vi "host.vi"() -> ()   [LabVIEW 2020]
uses:
  <vilib>/FPGAPlugInAG/cRIO-9035/niLvFpga_Open_cRIO-9035.vi
  <vilib>/rvi/interface/common/dynamic/niFpgaDynamicAddResources.vi
  <vilib>/Utility/error.llb/Error Cluster From Error Code.vi
  <vilib>/rvi/errors/niLvFpgaAdjustHostInterfaceError.vi
  <vilib>/FPGAPlugInAG/Dynamic/niLvFpga_Run_Dynamic.vi
  <vilib>/FPGAPlugInAG/Dynamic/niLvFpga_Close_Dynamic.vi
  <vilib>/rvi/interface/nirviOpenFPGA/nirviOpenFPGA.xnode
  FPGA Bitfiles/v1.2_FPGATarget_target_ruB+bBOu3LI.lvbitx
  target.vi
  <vilib>/rvi/interface/nirviMethod/nirviMethod.xnode
  <vilib>/rvi/interface/nirviReadWriteControl/nirviReadWriteControl.xnode
  <vilib>/rvi/interface/nirviCloseFPGA/nirviCloseFPGA.xnode
  <vilib>/rvi/errors/niLvFpgaMergeErrorWithErrorCode.vi
  <vilib>/FPGAPlugInAG/Dynamic/niLvFpga_WriteFifo_Dynamic.vi
  <vilib>/FPGAPlugInAG/Dynamic/niLvFpga_ReadFifo_Dynamic.vi
  NiFpgaLv.dll
  <vilib>/rvi/interface/Simulation/niFpgaSimulationCallBeginRW.vi
panel:
  out "transposed array":fxp<+/-,32,16>[][](array[numeric])
  out "output array":fxp<+/-,32,16>[][](array[numeric])
  out "n out":i32
  out "m out":i32
  out "sum of error":dbl
  out "B - FPGA code":sgl[][](array[numeric])
  out "A":sgl[][](array[numeric])
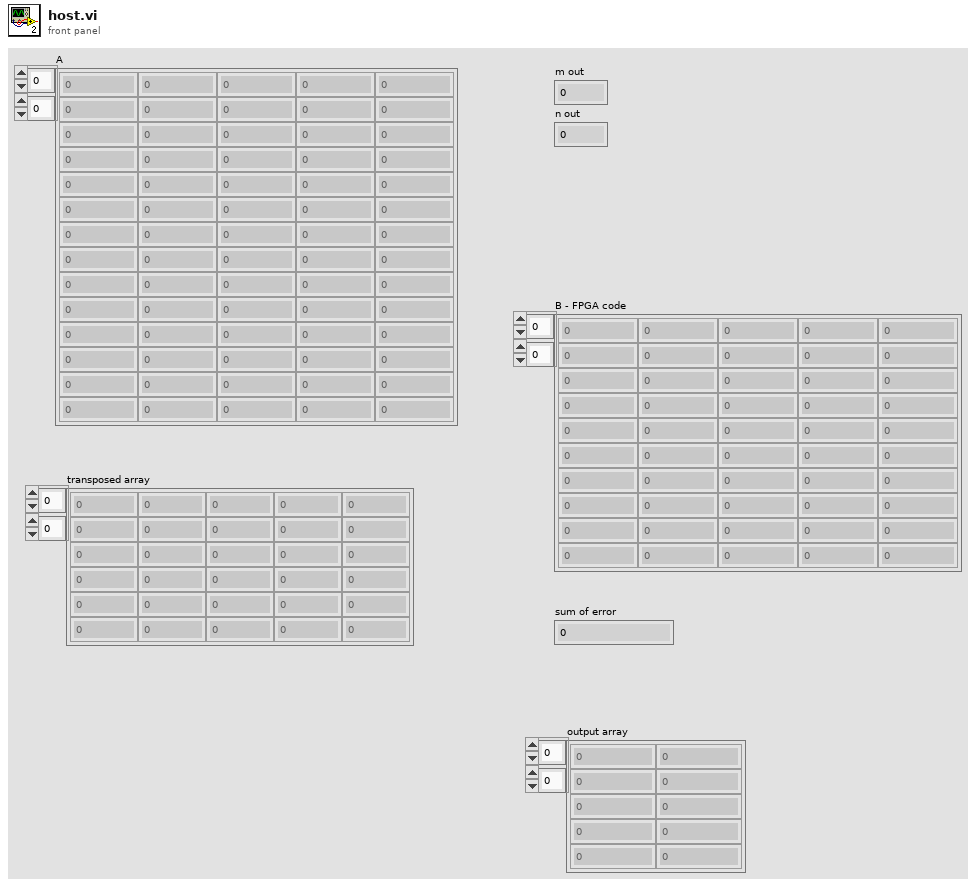
[diagram p1: front panel]
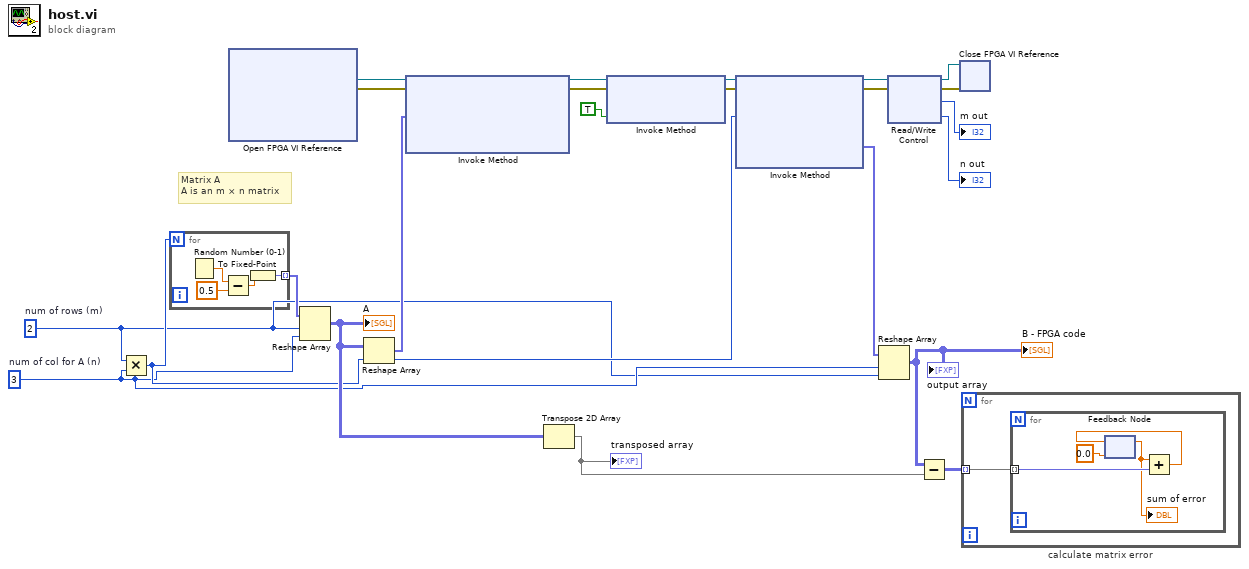
[diagram p0: block diagram]
diagram:
  w8 = 3  # num of col for A (n)
  w7 = 2  # num of rows (m)
  # "Matrix A\nA is an m × n matrix"
  n1 = Multiply(x=w7, y=w8) -> (x*y=w12:i32)
  n2 = for {
    N: w12 -> [_]
    tunnel: [w25] -> w18 mode=indexing
    n3 = Random Number (0-1)() -> (number: 0 to 1=w27:dbl)
    n4 = Subtract(x=w27, y=sgl 0.5) -> (x-y=w24:sgl)
    n5 = To Fixed-Point(number=w24) -> (fixed-point=w25:fxp<+/-,32,16>)  [unwired: 1 in]
  }
  n6 = xnode "Open FPGA VI Reference"() -> ("FPGA VI Reference Out"=w22:refnum<k20>, "error out"=w21:errorcluster)  [unwired: 2 in]
  n7 = Reshape Array(w18, w7, w8) -> (w14:fxp<+/-,32,16>[][])
  "A" <- w14
  n8 = Reshape Array(w14, w12) -> (w17:fxp<+/-,32,16>[])
  n9 = xnode "Invoke Method"("FPGA VI Reference In"=w22, "error in"=w21, "Data"=w17) -> ("FPGA VI Reference Out"=w11:refnum<k20>, "error out"=w10:errorcluster)  [unwired: 1 in, 1 out]
  n10 = Transpose 2D Array(2D array=w14) -> (transposed array=w13:fxp<+/-,32,16>[][])
  "transposed array" <- w13
  n11 = xnode "Invoke Method"("FPGA VI Reference In"=w11, "error in"=w10, "Wait Until Done (F)"=TRUE) -> ("FPGA VI Reference Out"=w20:refnum<k20>, "error out"=w19:errorcluster)
  n12 = xnode "Invoke Method"("FPGA VI Reference In"=w20, "error in"=w19, "Number of Elements"=w12) -> ("FPGA VI Reference Out"=w6:refnum<k20>, "error out"=w2:errorcluster, "Data"=w15:fxp<+/-,32,16>[])  [unwired: 1 in, 1 out]
  n13 = Reshape Array(w15, w8, w7) -> (w9:fxp<+/-,32,16>[][])
  "B - FPGA code" <- w9
  "output array" <- w9
  n14 = xnode "Read/Write Control"("FPGA VI Reference In"=w6, "error in"=w2) -> ("FPGA VI Reference Out"=w3:refnum<k20>, "error out"=w1:errorcluster, "m"=→"m out":i32, "n"=→"n out":i32)
  n15 = Subtract(x=w9, y=w13) -> (x-y=w16:fxp<+/-,33,17>[][])
  n16 = xnode "Close FPGA VI Reference"("FPGA VI Reference In"=w3, "error in"=w1) -> ()  [unwired: 1 out]
  n17 = for "calculate matrix error" {
    tunnel: w16 -> [w28] mode=indexing
    n18 = for {
      tunnel: w28 -> [w32] mode=indexing
      n19 = feedback #1(0.0) -> (w30:dbl)
      "sum of error" <- w30
      n20 = Add(x=w30, y=w32) -> (x+y=w31:dbl)
      n21 = feedback-in #1(w31) -> ()
    }
  }
